vi "Sift Create Ingestion Config.vi"(6 "Asset Name":string, 7 "Channel Name Prefix":string, 8 "error in (no error)":errorcluster, 9 "Data to Write In":cluster{variant[], string[]}, 10 "Old Stream Names":string[](array[string]), 11 "Sift Client in":refnum<class "Sift Client.lvclass">) -> (0 "error out":errorcluster, 3 "Sift Client out":refnum<class "Sift Client.lvclass">)   [LabVIEW 2024, in "Sift Stream.lvlib" / "Sift Stream.lvclass"]
doc: "Create a Sift ingestion config on initial running or if the channels have changed."
uses:
  Sift Stream.lvclass
  Sift Stream.lvclass/Sift Stream.ctl
  <vilib>/Sift/Sift/Sift API/Types/Data Type.ctl
  <vilib>/Sift/Sift/Sift Client.lvlib
  <userlib>/_OpenG.lib/string/string.llb/openg_string.lvlib
  <vilib>/Utility/Data Type/NI_Data Type.lvlib
  <vilib>/Sift/Sift/Sift API/Sift Client.lvclass
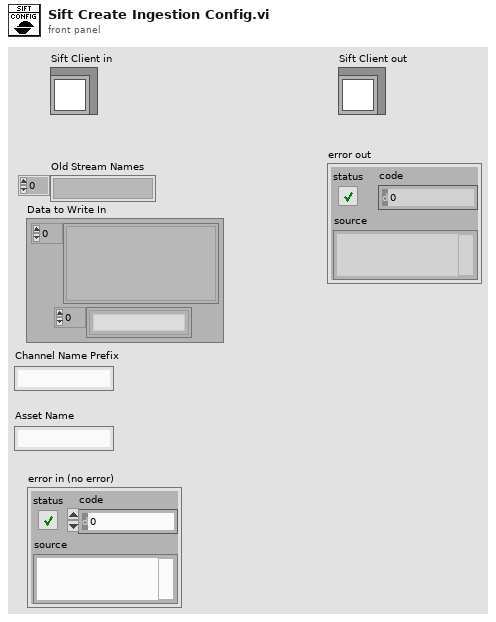
[diagram p1: front panel]
types:
  T1 = typedef "Sift Client.lvlib/Data Type.ctl" = enum8{"double", "float", "uint64", "int64", "uint32", "int32", "bool", "enum", "string"}
  T2 = typedef "NI_Data Type.lvlib/Data Type.ctl" = enum8{"Invalid Type", "Void", "I8", "I16", "I32", "I64", "U8", "U16", "U32", "U64", "Single Float", "Double Float", "Extended Float", "Single Complex", "Double Complex", "Extended Complex", "Enum U8", "Enum U16", "Enum U32", "Enum U64", "Single Float With Unit", "Double Float With Unit", "Extended Float With Unit", "Single Complex with Unit", "Double Complex with Unit", "Extended Complex with Unit", "Boolean", "String", "Path", "Picture", "Tag", "Array", "Cluster", "Variant", "LV Variant", "Waveform", "Timestamp", "Digital Waveform", "Digital Data", "ExpressData", "Refnum", "External Data", "VI", "Poly VI", "LabVIEW Class Instance", "Fixed Point", "Set Collection", "Map Collection"}
  T3 = typedef "Sift Client.lvlib/Channel Config.ctl" = cluster{"name":string, "data_type":T1, "description":string, "component":string, "unit":string, "bit_field_elements":T4[], "enum_types":T5[]}
  T4 = typedef "Bit Field.ctl" = cluster{"index":u32, "bit_count":u32, "name":string}
  T5 = typedef "Sift Client.lvlib/Enum.ctl" = cluster{"key":u32, "name":string}
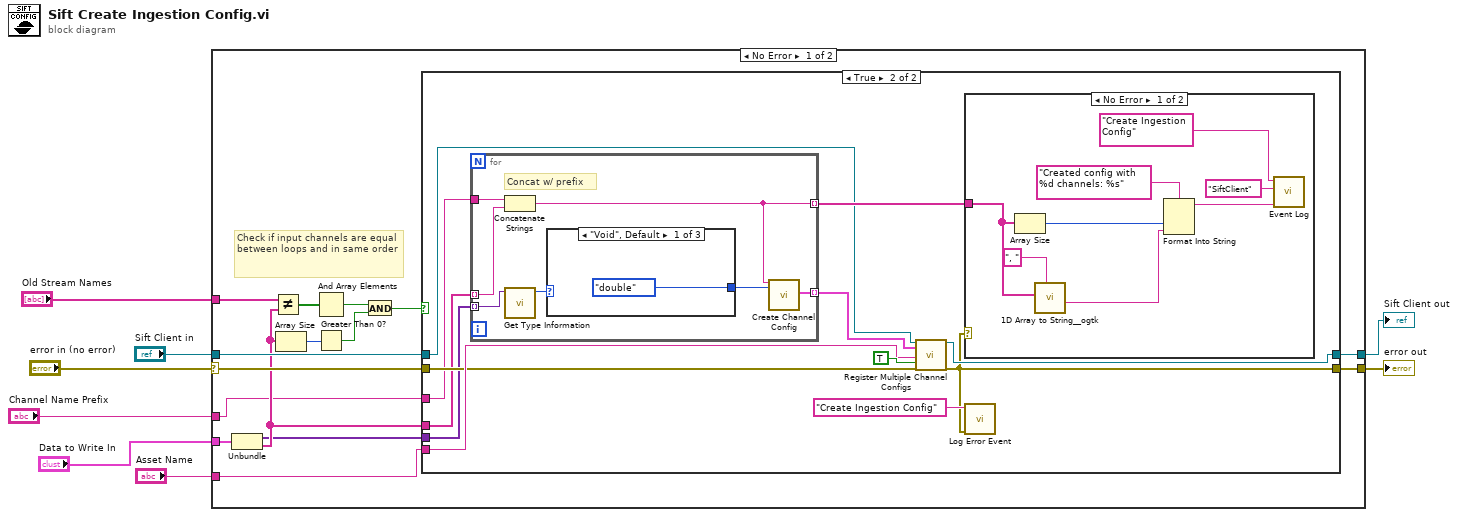
[diagram p0: block diagram]
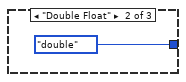
[diagram p4: hidden frame]
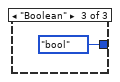
[diagram p5: hidden frame]
diagram:
  n1 = case shown="No Error" "error in (no error)" {
    selector: "error in (no error)" -> [w13 w56]
    tunnel: [w23 w57] -> w8
    tunnel: "Sift Client in" -> [w22 w57]
    tunnel: "Old Stream Names" -> [w21 _]
    tunnel: [w19 w56] -> w5
    tunnel: "Asset Name" -> [w18 _]
    tunnel: "Data to Write In" -> [w12 _]
    tunnel: "Channel Name Prefix" -> [w9 _]
    frame No Error {
      # "Check if input channels are equal between loops and in same order"
      n2 = Unbundle(w12) -> (w10:variant[], w11:string[])
      n3 = Not Equal?(x=w21, y=w11) -> (x != y?=w20:bool[])
      n4 = Array Size(array=w11) -> (size(s)=w17:i32)
      n5 = And Array Elements(Boolean array=w20) -> (logical AND=w16:bool)
      n6 = Greater Than 0?(x=w17) -> (x > 0?=w15:bool)
      n7 = And(x=w16, y=w15) -> (x .and. y?=w14:bool)
      n8 = case shown="True" w14 {
        tunnel: w22 -> [w25 w26]
        tunnel: [w24 w29] -> w19
        tunnel: [w25 w36] -> w23
        tunnel: w18 -> [_ w34]
        tunnel: w11 -> [_ w32]
        tunnel: w13 -> [w24 w33]
        tunnel: w9 -> [_ w28]
        tunnel: w10 -> [_ w27]
        frame False {
        }
        frame True {
          n9 = for {
            tunnel: [w52] -> w37 mode=indexing
            tunnel: w32 -> [w49] mode=indexing
            tunnel: [w48] -> w31 mode=indexing
            tunnel: w28 -> [w50]
            tunnel: w27 -> [w47] mode=indexing
            # "Concat w/ prefix"
            n10 = Concatenate Strings(w50, w49) -> (w48:string)
            n11 = call <vilib>:"Get Type Information.vi"("variant"=w47) -> ("type"=w46:T2)  [unwired: 6 in, 4 out]
            n12 = case shown="\"Void\", Default" w46 {
              tunnel: [Data_Type."double" ("Enum") Data_Type."double" ("Enum") Data_Type."bool" ("Enum")] -> w51
              frame "Void", Default {
              }
              frame "Double Float" {
              }
              frame "Boolean" {
              }
            }
            n13 = call <vilib>:"Create Channel Config.vi"("Name"=w48, "Data Type"=w51) -> ("Output"=w52:T3)  [unwired: 17 in]
          }
          n14 = call-dynamic "Register Multiple Channel Configs.vi"("Sift Client in"=w26, "Channel Configs"=w37, "Asset Name"=w34, "Submit Ingestion Config"=TRUE, "error in (no error)"=w33) -> ("Sift Client out"=w36:refnum<class "Sift Client.lvclass">, "error out"=w29:errorcluster)  [unwired: 12 in, 1 out]
          n15 = case shown="No Error" w29 {
            tunnel: w31 -> [w38 _]
            frame No Error {
              n16 = Array Size(array=w38) -> (size(s)=w45:i32)
              n17 = call <userlib>:"1D Array to String__ogtk.vi"("delimiter (Tab)"=", ", "Array of Strings"=w38) -> ("delimited string"=w44:string)  [unwired: 9 in]
              n18 = Format Into String(format string="Created config with %d channels: %s", w45, w44) -> (resulting string=w43:string)  [unwired: 2 in, 1 out]
              n19 = call "Event Log.vi"("Message"=w43, "Event Type"="SiftClient", "Location"="Create Ingestion Config") -> ()  [unwired: 9 in]
            }
            frame Error {
            }
          }
          n20 = call "Log Error Event.vi"("error in (no error)"=w29, "Location"="Create Ingestion Config") -> ()  [unwired: 10 in]
        }
      }
    }
    frame Error {
    }
  }
  "Sift Client out" <- w8
  "error out" <- w5
